vi "File Path Functional Global.vi"(9 "Enum":enum16{"Get Data", "Set Data"}(ring), 11 "File Path Control":path) -> (3 "File Path Output":path)   [LabVIEW 2014]
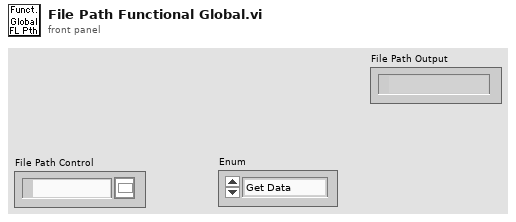
[diagram p1: front panel]
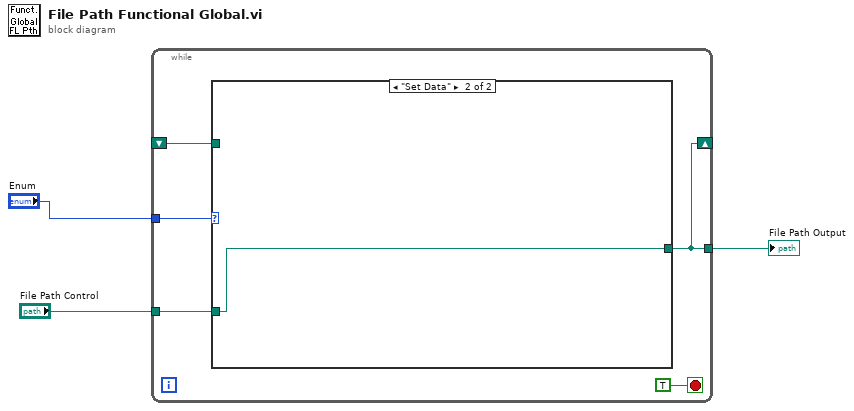
[diagram p0: block diagram]
diagram:
  n1 = while {
    tunnel: "Enum" -> [w8]
    shift-right: [w5] -> _
    shift-left: _ -> [w4]
    tunnel: "File Path Control" -> [w6]
    tunnel: [w5] -> w1
    stop <- TRUE stop-if-true
    n2 = case shown="\"Set Data\"" w8 {
      tunnel: w6 -> [_ w10]
      tunnel: [w9 w10] -> w5
      tunnel: w4 -> [w9 _]
      frame "Get Data", Default {
      }
      frame "Set Data" {
      }
    }
  }
  "File Path Output" <- w1
